vi "sub_950-item-parsing-raw.vi"(11 "items":dbl[][](array[numeric])) -> ()   [LabVIEW 2019]
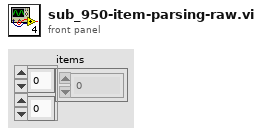
[diagram p1: front panel]
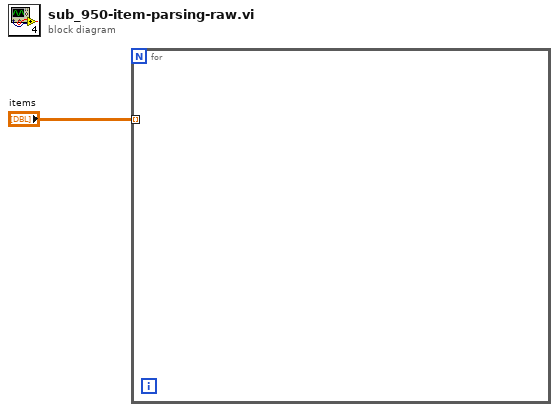
[diagram p0: block diagram]
diagram:
  n1 = for {
    tunnel: "items" -> [_] mode=indexing
  }
